vi "Read gas bag Arduino.vi"(0 "Sensor configuration":T1, 3 "Error In":errorcluster) -> (7 "Data":dbl[](array[numeric]), 8 "Names":string[](array[string]), 9 "Communication error":string, 10 "Error Out":errorcluster)   [LabVIEW 2015]
uses:
  Sensor configuration.ctl
  Channel type.ctl
  <vilib>/Utility/error.llb/DialogType.ctl
panel:
  out "number":i32
  out "output string":string
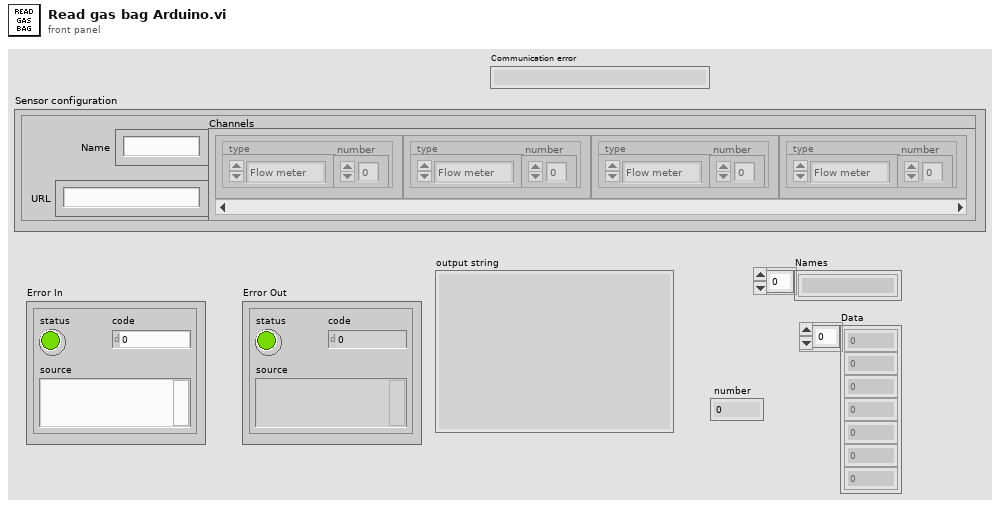
[diagram p1: front panel]
types:
  T1 = typedef "Sensor configuration.ctl" = cluster{"Name":string, "URL":string, "Channels":cluster{"type":T2, "number":dbl}[]}
  T2 = typedef "Channel type.ctl" = enum16{"Volts", "Flow meter", "Tank pressure", "Dewar level", "Raw ADC"}
  T3 = typedef "DialogType.ctl" = u16
  T4 = enum16{"Read", "Write", "ReadWrite", "BufferedRead", "BufferedReadWrite"}
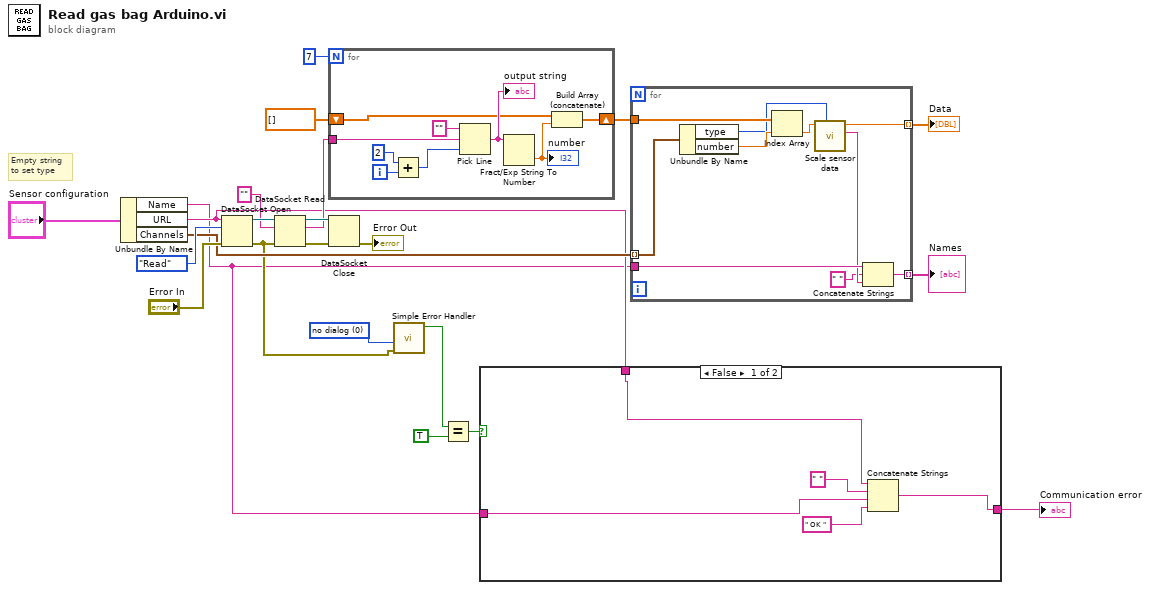
[diagram p0: block diagram]
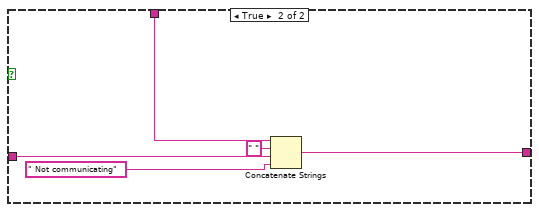
[diagram p2: hidden frame]
diagram:
  w7 = T3 0 items=["no dialog", "OK message", "continue or stop message", "OK message + warnings", "continue/stop + warnings"] ("type of dialog (OK msg:1)")
  # "Empty string\nto set type"
  n1 = Unbundle By Name("Sensor configuration") -> ("Name"=w2:string, "URL"=w3:string, "Channels"=w12:cluster{"type":T2, "number":dbl}[])
  n2 = DataSocket Open(8:"Error In", 10:T4."Read" ("mode"), 11:w3) -> (0:w8:errorcluster, 3:w23:refnum<k13>)  [unwired: 1 in]
  n3 = DataSocket Read(8:w8, 10:"", 11:w23) -> (0:w21:errorcluster, 2:w18:string, 3:w22:refnum<k13>)  [unwired: 2 in, 4 out]
  n4 = for {
    N: 7 -> [_]
    tunnel: w18 -> [w32]
    shift-right: [w28] -> w11
    shift-left: dbl[] [] -> [w27]
    i -> [w29]
    n5 = Add(x=2, y=w29) -> (x+y=w25:i32)
    n6 = Pick Line(string ("")="", multi-line string=w32, line index=w25) -> (output string=w30:string)
    "output string" <- w30
    n7 = Fract/Exp String To Number(string=w30) -> (number=w26:dbl)  [unwired: 3 in, 1 out]
    "number" <- w26
    n8 = Build Array (concatenate)(w27, w26) -> (w28:dbl[])
  }
  n9 = DataSocket Close(8:w21, 11:w22) -> (0:→"Error Out":errorcluster)  [unwired: 1 in, 1 out]
  n10 = call <vilib>:"Simple Error Handler.vi"("type of dialog (OK msg:1)"=w7, "error in (no error)"=w8) -> ("error?"=w5:bool)  [unwired: 3 in, 4 out]
  n11 = Equal?(x=w5, y=TRUE) -> (x = y?=w6:bool)
  n12 = case shown="False" w6 {
    tunnel: w3 -> [w35 w40]
    tunnel: w2 -> [w33 w41]
    tunnel: [w37 w38] -> w1
    frame False {
      n13 = Concatenate Strings(w35, " " ("string"), w33, " OK ") -> (w37:string)
    }
    frame True {
      n14 = Concatenate Strings(w40, " " ("string"), w41, " Not communicating" ("Message")) -> (w38:string)
    }
  }
  "Communication error" <- w1
  n15 = for {
    tunnel: w12 -> [w52] mode=indexing
    tunnel: w11 -> [w50]
    tunnel: [w47] -> w10 mode=indexing
    tunnel: w2 -> [w46]
    tunnel: [w43] -> w9 mode=indexing
    n16 = Unbundle By Name(w52) -> ("type"=w48:T2, "number"=w51:dbl)
    n17 = Index Array(array=w50, index=w51) -> (element=w49:dbl)
    n18 = call "Scale sensor data.vi"("Channel type"=w48, "RAW Value"=w49) -> ("Type name"=w45:string, "Scaled value"=w47:dbl)  [unwired: 8 in]
    n19 = Concatenate Strings(w46, " " ("string"), w45) -> (w43:string)
  }
  "Data" <- w10
  "Names" <- w9
